vi "SATTdll_d.vi"(7 "Refpropdllpath":path, 8 "error in (no error)":errorcluster, 9 "Component Molar Fractions":dbl[](array[numeric])=[1.0, 0.0, 0.0, 0.0, 0.0, 0.0, 0.0, 0.0, 0.0, 0.0, 0.0, 0.0, 0.0, 0.0, 0.0, 0.0, 0.0, 0.0, 0.0, 0.0], 10 "i":dbl, 11 "Temp (deg C)":dbl=30.0) -> (0 "error out":errorcluster, 3 "tdataout":dbl[](array[numeric]), 4 "dll_path_out":path)   [LabVIEW 2017]
doc: "Calculate for saturated liquid and vapor states given temperature and the composition of one phase\n\n inputs:\n t--temperature [K]\n x--composition [array of mol frac] (phase specified by kph)\n kph--phase flag: 1 = input x is liquid composition (bubble point)\n 2 = input x is vapor composition (dew point)\n 3 = input x is liquid comp (freezing point)\n 4 = input x is vapor comp (sublimation point)\n outputs:\n p--pressure [kPa]\n rhol--molar density [mol/L] of saturated liquid\n rhov--molar density [mol/L] of saturated vapor\n xliq--liquid phase composition [array of mol frac]\n xvap--vapor phase composition [array of mol frac]\n ierr--error flag: 0 = successful\n 1 = T < Tmin\n 8 = x out of range\n 9 = T and x out of range\n 120 = CRITP did not converge\n 121 = T > Tcrit\n 122 = TPRHO-liquid did not converge (pure fluid)\n 123 = TPRHO-vapor did not converge (pure fluid)\n 124 = pure fluid iteration did not converge\n following 3 error codes are advisory--iteration will either\n converge on later guess or error out (ierr = 128)\n -125 = TPRHO did not converge for parent ph (mix)\n -126 = TPRHO did not converge for incipient (mix)\n -127 = composition iteration did not converge\n 128 = mixture iteration did not converge\n herr--error string if ierr<>0 (character*255)"
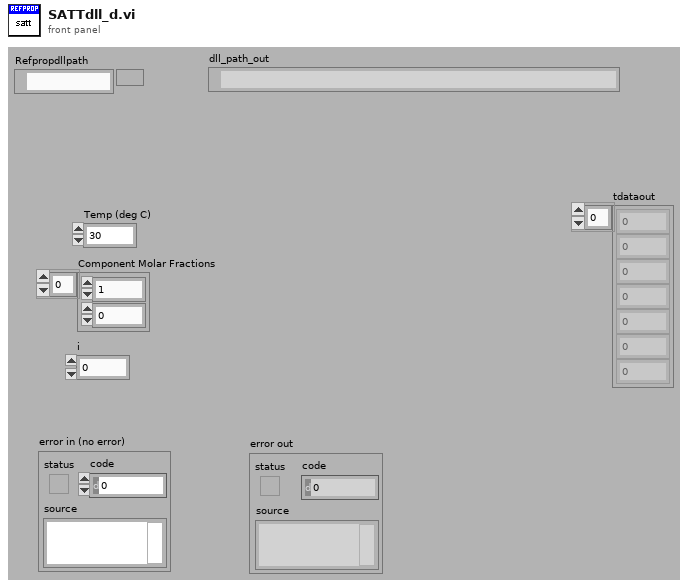
[diagram p1: front panel]
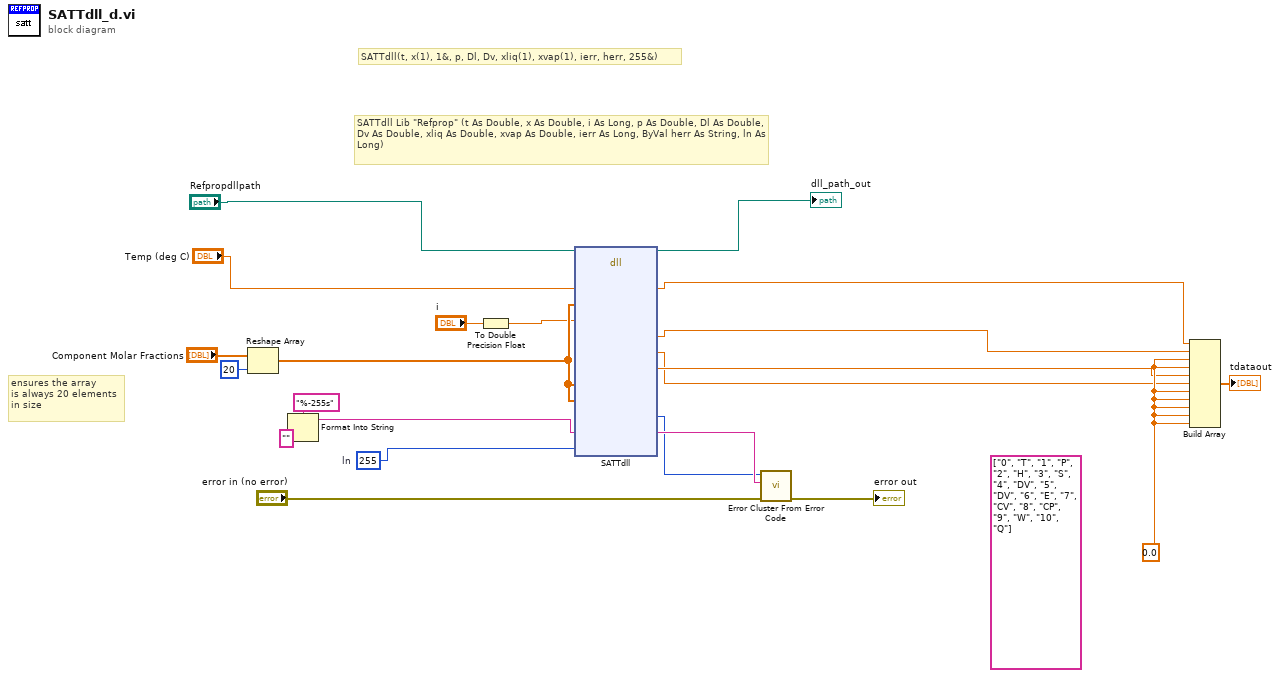
[diagram p0: block diagram]
diagram:
  (unwired) string[][] [["0", "T"], ["1", "P"], ["2", "H"], ["3", "S"], ["4", "DV"], ["5", "DV"], ["6", "E"], ["7", "CV"], ["8", "CP"], ["9", "W"], ["10", "Q"]] ("数组")
  w6 = 0.0 ("h")
  w12 = 255  # ln
  # "SATTdll Lib \"Refprop\" (t As Double, x As Double, i As Long, p As Double, Dl As Double, Dv As Double, xliq As Double, xvap As Double, ierr As Long, ByVal herr As String, ln As Long)"
  # "SATTdll(t, x(1), 1&, p, Dl, Dv, xliq(1), xvap(1), ierr, herr, 255&)"
  # "ensures the array\nis always 20 elements\nin size"
  n1 = Reshape Array("Component Molar Fractions", 20 ("dimension size")) -> (w19:dbl[])
  n2 = Format Into String(format string="%-255s", "") -> (resulting string=w11:string)  [unwired: 2 in, 1 out]
  n3 = To Double Precision Float(number="i") -> (double precision float=w15:dbl)
  n4 = dll-call lib="refprop.DLL" fn="SATTdll" label="sattDLL"(path in="Refpropdllpath", "t"="Temp (deg C)", "x"=w19, "i"=w15, "xliq"=w19, "xvap"=w19, "herr"=w11, "ln"=w12) -> (path out=→"dll_path_out":path, "t"=w5:dbl, "p"=w7:dbl, "Dl"=w3:dbl, "Dv"=w4:dbl, "ierr"=w13:i32, "herr"=w14:string)  [unwired: 12 in, 1 out]
  n5 = call <vilib>:"Error Cluster From Error Code.vi"("error in (no error)"="error in (no error)", "error message (\"\")"=w14, "error code (0)"=w13) -> ("error out"=→"error out":errorcluster)  [unwired: 6 in]
  n6 = Build Array(w5, w7, w6, w6, w4, w3, w6, w6, w6, w6, w6) -> (→"tdataout":dbl[])
